vi "4 Tap 12-Bit.vi"() -> (0 "PixelData":T1)   [LabVIEW 2016]
uses:
  <vilib>/rvi/eio/common/nirviEmuTemplateMethod_errors.vi
  <vilib>/eio/EIONode/EIONode.xnode
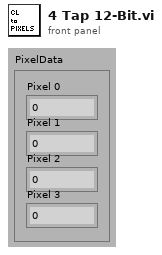
[diagram p1: front panel]
types:
  T1 = cluster{"Pixel 0":u16, "Pixel 1":u16, "Pixel 2":u16, "Pixel 3":u16}
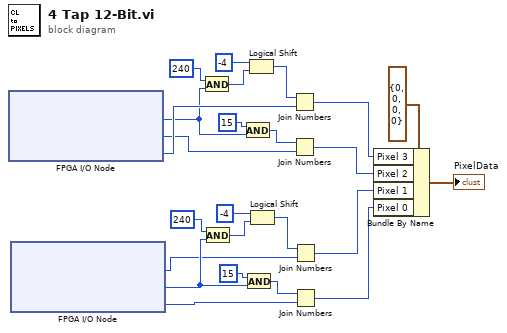
[diagram p0: block diagram]
diagram:
  n1 = xnode "FPGA I/O Node"() -> ("IO Module\\CL Port F"=w3:u8, "IO Module\\CL Port E"=w4:u8, "IO Module\\CL Port D"=w5:u8)  [unwired: 3 in, 3 out]
  n2 = xnode "FPGA I/O Node"() -> ("IO Module\\CL Port C"=w16:u8, "IO Module\\CL Port B"=w18:u8, "IO Module\\CL Port A"=w17:u8)  [unwired: 3 in, 3 out]
  n3 = And(x=u8 240 ("hi"), y=w3) -> (x .and. y?=w9:u8)
  n4 = And(x=u8 240 ("hi"), y=w18) -> (x .and. y?=w21:u8)
  n5 = And(x=u8 15 ("hi"), y=w3) -> (x .and. y?=w7:u8)
  n6 = And(x=u8 15 ("hi"), y=w18) -> (x .and. y?=w23:u8)
  n7 = Logical Shift(y=i8 -4, x=w9) -> (x << y=w11:u8)
  n8 = Logical Shift(y=i8 -4, x=w21) -> (x << y=w19:u8)
  n9 = Join Numbers(hi=w11, lo=w5) -> ((hi.lo)=w2:u16)
  n10 = Join Numbers(hi=w7, lo=w4) -> ((hi.lo)=w1:u16)
  n11 = Join Numbers(hi=w19, lo=w16) -> ((hi.lo)=w14:u16)
  n12 = Join Numbers(hi=w23, lo=w17) -> ((hi.lo)=w15:u16)
  n13 = Bundle By Name(cluster=T1 {"Pixel 0"=0, "Pixel 1"=0, "Pixel 2"=0, "Pixel 3"=0} ("PixelData"), "Pixel 3"=w2, "Pixel 2"=w1, "Pixel 1"=w14, "Pixel 0"=w15) -> (→"PixelData":T1)
